vi "SENS_IF_FILT_STAG_PAR.vi"(0 "VISA IN":refnum<visa-resource-name>, 1 "Filter Parameter":string, 2 "Parameter Value":string, 5 "error in":errorcluster, 7 "Channel":i32) -> (14 "VISA Out":refnum<visa-resource-name>, 19 "error out":errorcluster)   [LabVIEW 2018, in "PNA-X.lvlib"]
doc: "SENSe<cnum>:IF:FILTer:STAGe3:PARameter <p>, <value> \n(Read-Write) Sets and returns the Stage 3 filter parameters. \nMust first select the filter type (SENS:IF:FILT:STAGe3:TYPE) before setting these parameters \nUse SENSe:IF:FILT:STAGE3:PCAT? to return a list of the available parameters for the currently \nselected filter type. \nCritical Note \nParameters \n<cnum> Existing channel number. If unspecified, <cnum> is set to 1. \n<p> (String) Filter parameter. Choose from: \n\"C\" - Tap count (Tukey, RECT, PWIN) \n\"P\" - Period (PWIN ONLY) \n\"D\" - Delay (PWIN ONLY) \n\"W\" - Width (PWIN ONLY) \n\"R\" - Ramp Count (PWIN ONLY) \n1758\n\n<value> (String) Parameter Value for the specified stage 3 parameter. Use the query form \nto return the minimum and maximum values for the specified parameter. \nExamples SENS:IF:FILT:STAGe3:PAR \"C\",64 \nsense2:if:filter:stage3:parameter \"d\",0.5E-6 \nQuery Syntax SENSe<cnum>:IF:FILTer:STAGE3:PARameter? <p> \nreturns the current parameter value"
uses:
  PNA-X.lvlib
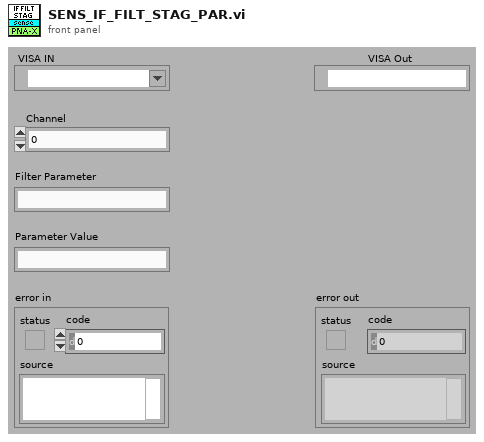
[diagram p1: front panel]
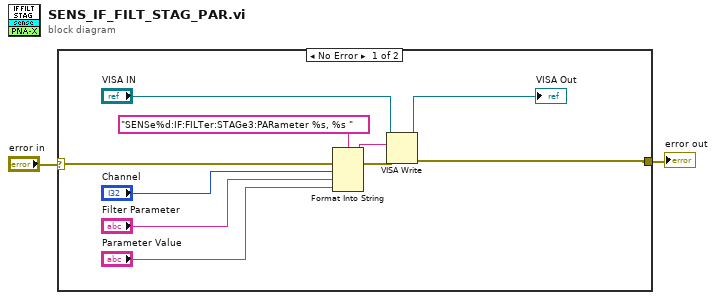
[diagram p0: block diagram]
diagram:
  n1 = case shown="No Error" "error in" {
    selector: "error in" -> [w12 w13]
    tunnel: [w7 w13] -> w1
    frame No Error {
      n2 = Format Into String(format string="SENSe%d:IF:FILTer:STAGe3:PARameter %s, %s " ("Cmdline"), error in=w12, "Channel", "Filter Parameter", "Parameter Value") -> (resulting string=w10:string, error out=w11:errorcluster)  [unwired: 1 in]
      n3 = VISA Write(VISA resource name="VISA IN", write buffer=w10, error in (no error)=w11) -> (VISA resource name out=→"VISA Out":refnum<visa-resource-name>, error out=w7:errorcluster)  [unwired: 1 out]
    }
    frame Error {
    }
  }
  "error out" <- w1
